vi "ButtonColorChooser.vi"(7 "Un-selected Color":cluster{u32, u32}[](array[cluster])=[{16773632, 16448250}, {16448250, 16448250}], 9 "Disallowed":bool, 10 "Confirmed":bool) -> (2 "Final Color":cluster{u32, u32}[](array[cluster]))   [LabVIEW 2019]
doc: "Allows GUI buttons to be colored by three different states: Pressed, Unpressed, and Disabled."
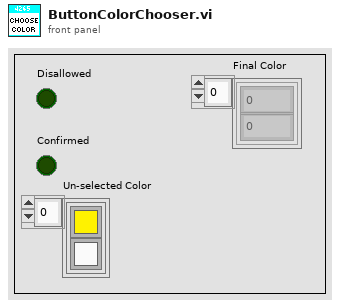
[diagram p1: front panel]
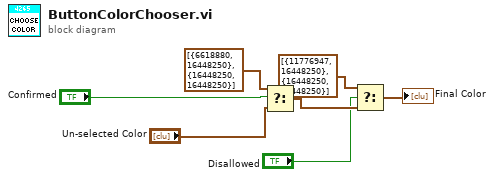
[diagram p0: block diagram]
diagram:
  n1 = Select(t=cluster{u32, u32}[] [{6618880, 16448250}, {16448250, 16448250}] ("Colors [4]"), s="Confirmed", f="Un-selected Color") -> (s? t:f=w4:cluster{u32, u32}[])
  n2 = Select(t=cluster{u32, u32}[] [{11776947, 16448250}, {16448250, 16448250}] ("Colors [4]"), s="Disallowed", f=w4) -> (s? t:f=→"Final Color":cluster{u32, u32}[])
